vi "Configure Frequency Sweep List .vi"(7 "Stop Frequency (5E+7 Hz)":dbl=50000000.0, 8 "error in (no error)":errorcluster, 9 "Start Frequency (5E+7 Hz)":dbl=50000000.0, 10 "Enable List Mode (F: Disable)":bool, 11 "VISA resource name":refnum<visa-resource-name>) -> (0 "error out":errorcluster, 3 "VISA resource name out":refnum<visa-resource-name>)   [LabVIEW 2018, in "Agilent U2000 Series.lvlib"]
doc: "Configures frequency sweep list.\n\nNote: \nThis VI is only applicable for U2040 X-Series."
uses:
  Agilent U2000 Series.lvlib
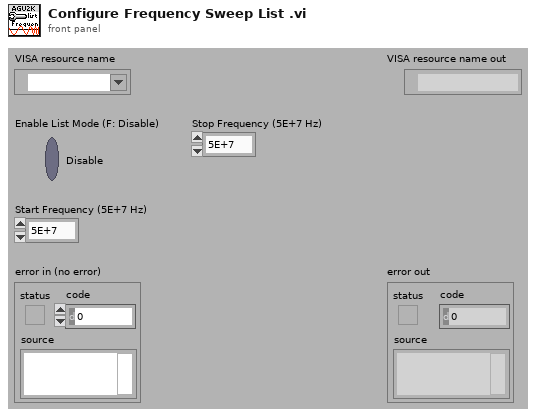
[diagram p1: front panel]
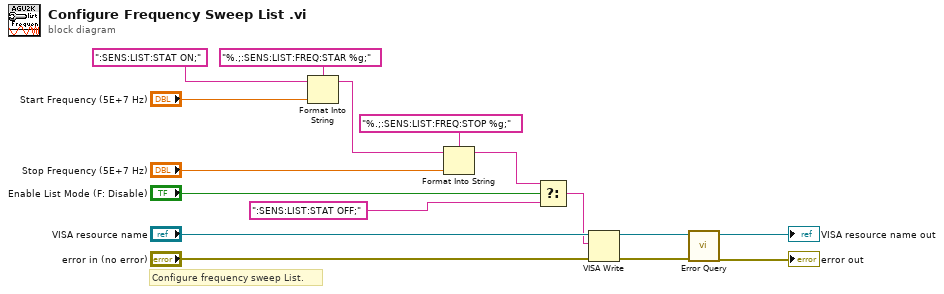
[diagram p0: block diagram]
diagram:
  # "Configure frequency sweep List."
  n1 = Format Into String(format string="%.;:SENS:LIST:FREQ:STAR %g;", initial string=":SENS:LIST:STAT ON;", "Start Frequency (5E+7 Hz)") -> (resulting string=w2:string)  [unwired: 1 in, 1 out]
  n2 = Format Into String(format string="%.;:SENS:LIST:FREQ:STOP %g;", initial string=w2, "Stop Frequency (5E+7 Hz)") -> (resulting string=w1:string)  [unwired: 1 in, 1 out]
  n3 = Select(t=w1, s="Enable List Mode (F: Disable)", f=":SENS:LIST:STAT OFF;") -> (s? t:f=w4:string)
  n4 = VISA Write(VISA resource name="VISA resource name", write buffer=w4, error in (no error)="error in (no error)") -> (VISA resource name out=w10:refnum<visa-resource-name>, error out=w9:errorcluster)  [unwired: 1 out]
  n5 = call "Error Query.vi"("error in (no error)"=w9, "VISA resource name"=w10) -> ("error out"=→"error out":errorcluster, "VISA resource name out"=→"VISA resource name out":refnum<visa-resource-name>)  [unwired: 6 in, 2 out]
